vi "MinMax Decimation.vi"(10 "Params":T1, 11 "XY Data":cluster{"X":dbl[], "Y":dbl[]}[](array[cluster])) -> (3 "MinMax Data":cluster{dbl[], dbl[]}[](array[cluster]))   [LabVIEW 2020, in "VolatusGUIElements.lvlib"]
uses:
  VolatusGUIElements.lvlib
  Decimation Params.ctl
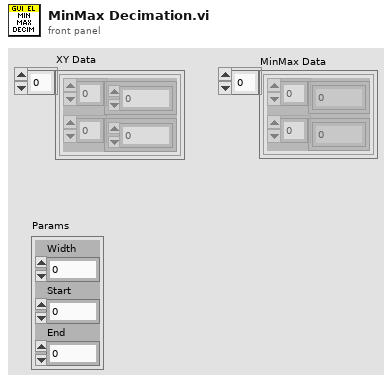
[diagram p1: front panel]
types:
  T1 = typedef "VolatusGUIElements.lvlib/Decimation Params.ctl" = cluster{"Width":i32, "Start":dbl, "End":dbl}
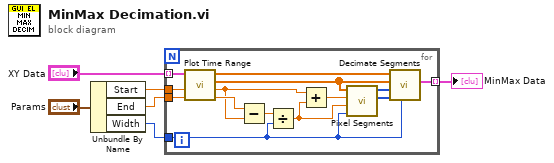
[diagram p0: block diagram]
diagram:
  n1 = Unbundle By Name("Params") -> ("Start"=w2:dbl, "End"=w1:dbl, "Width"=w4:i32)
  n2 = for {
    tunnel: w2 -> [w13]
    tunnel: w1 -> [w14]
    tunnel: "XY Data" -> [w20] mode=indexing
    tunnel: w4 -> [w11]
    tunnel: [w15] -> w3 mode=indexing
    n3 = call "Plot Time Range.vi"("End"=w14, "Start"=w13, "Plot Data"=w20) -> ("Actual End"=w8:dbl, "Actual Start"=w7:dbl, "X"=w18:dbl[], "Y"=w19:dbl[])  [unwired: 5 in]
    n4 = Subtract(x=w8, y=w7) -> (x-y=w12:dbl)
    n5 = Divide(x=w12, y=w11) -> (x/y=w9:dbl)
    n6 = Add(x=w7, y=w9) -> (x+y=w10:dbl)
    n7 = call "Pixel Segments.vi"("# px"=w11, "ds / px"=w9, "End of First px"=w10, "X"=w18) -> ("px Lengths"=w16:i32[], "px Starts"=w17:i32[])  [unwired: 6 in]
    n8 = call "Decimate Segments.vi"("Width"=w11, "px Lengths"=w16, "px Starts"=w17, "X"=w18, "Y"=w19) -> ("Decimated Data"=w15:cluster{"X":dbl[], "Y":dbl[]})  [unwired: 6 in]
  }
  "MinMax Data" <- w3
